vi "Setup Test Log.vi"(8 "error in (no error)":errorcluster, 10 "Model in":refnum<class "Model.lvclass">, 11 "Boot Loader in":refnum<class "Boot Loader.lvclass">) -> (0 "error out":errorcluster, 2 "Model out":refnum<class "Model.lvclass">, 3 "Boot Loader out":refnum<class "Boot Loader.lvclass">)   [LabVIEW 2015, in "Boot Loader.lvclass"]
uses:
  Boot Loader.lvclass
  Model/Model.lvclass
  Typedefs/Test Log Types.ctl
  Test Log/Test Log Factory/Test Log Factory.lvclass
  Model/Model.lvclass/Model.ctl
  Typedefs/FAMT Typedefs.lvlib
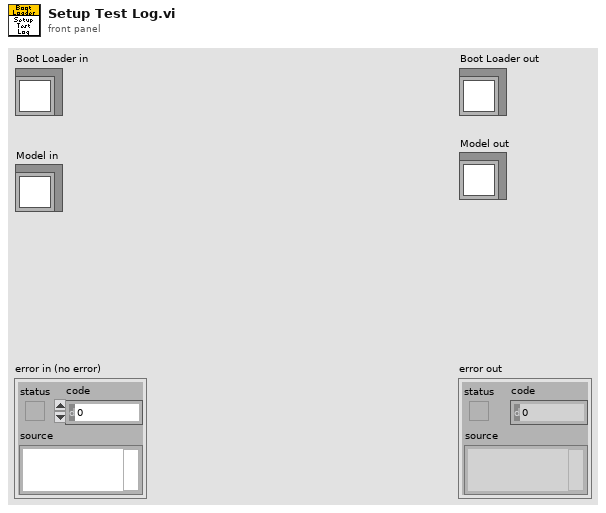
[diagram p1: front panel]
types:
  T1 = typedef "FAMT Typedefs.lvlib/Test Log Types.ctl" = enum16{"CSV Test Log"}
  T2 = typedef "FAMT Typedefs.lvlib/Scan Settings.ctl" = cluster{"Operator":string, "Scan Name":string, "Notes":string, "Axial Settings":T3, "Lateral Settings":T3, "Actuator Serial Number":string, "Actuator Orientation":string, "Actuator Inclination":string, "Test Stand Serial Number":string, "Operating Temperature":string, "Test Name":string}
  T3 = typedef "FAMT Typedefs.lvlib/Waveform Settings.ctl" = cluster{"Sample Count":u32, "Amplitude":dbl, "Offset":dbl, "Frequency":dbl[unit], "Waveform":T4, "F1":dbl[unit], "F2":dbl[unit], "Duty Cycle":dbl, "ILC Rate":dbl[unit], "Ramp Time":dbl[unit], "Hold Time":dbl[unit], "Settling Time":dbl[unit], "Delay":dbl[unit]}
  T4 = typedef "FAMT Typedefs.lvlib/Waveform Types.ctl" = enum16{"Sine", "Triangle", "Square", "Sawtooth", "Chirp", "Gaussian", "Trapezoid", "Constant"}
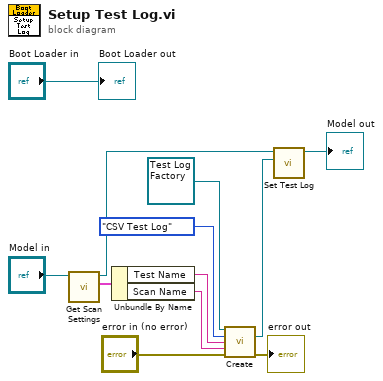
[diagram p0: block diagram]
diagram:
  n1 = call "Get Scan Settings.vi"("Model in"="Model in") -> ("Scan Settings"=w8:T2, "Model out"=w5:refnum<class "Model.lvclass">)  [unwired: 9 in]
  n2 = Unbundle By Name(w8) -> ("Test Name"=w2:string, "Scan Name"=w1:string)
  n3 = call-dynamic "Create.vi"("Test Log Factory in"=refnum<class "Test Log Factory.lvclass"> refnum ("Test Log Factory.lvclass"), "Test Log Types"=Test_Log_Types."CSV Test Log" ("TestLogTypes"), "Test Name"=w2, "Scan Name"=w1, "error in (no error)"="error in (no error)") -> ("Test Log"=w11:refnum<class "Test Log.lvclass">, "error out"=→"error out":errorcluster)  [unwired: 8 in, 1 out]
  n4 = call "Set Test Log.vi"("ITestLog.lvclass"=w11, "Model in"=w5) -> ("Model out"=→"Model out":refnum<class "Model.lvclass">)  [unwired: 9 in]
  "Boot Loader out" <- "Boot Loader in"
